vi "STS Calculator.vi"(8 "NumPts":i32=3, 10 "Saturation Id":dbl[](array[numeric]), 11 "Vg Column":dbl[](array[numeric])) -> (0 "STS Index":dbl, 2 "XY Graph":cluster{dbl[], dbl[]}[](graph), 3 "Sub Threshold Swing":dbl, 5 "Used Points":cluster{"Vg Used":dbl[], "Id Used":dbl[]})   [LabVIEW 2012]
uses:
  <vilib>/Analysis/NI_AALPro.lvlib
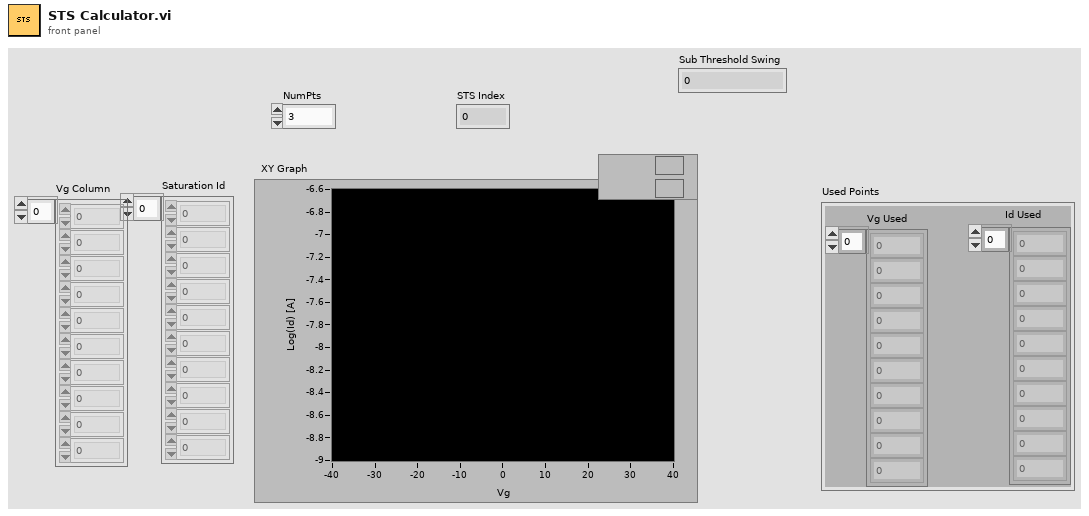
[diagram p1: front panel]
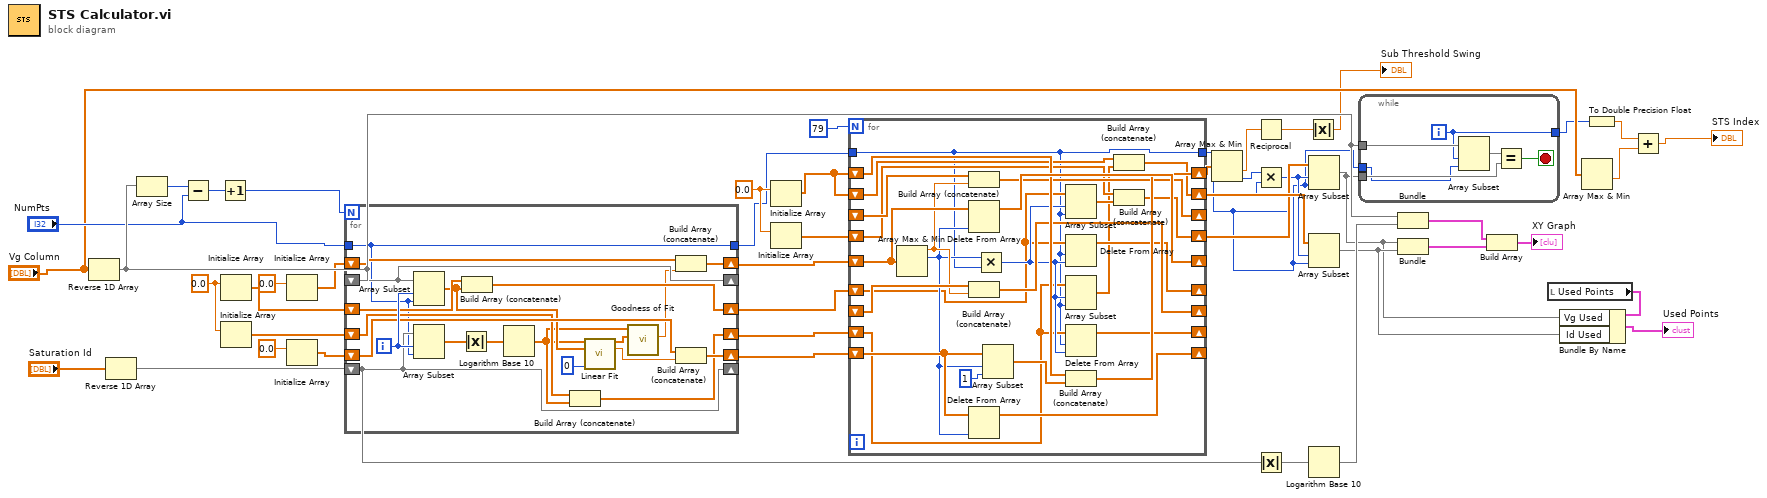
[diagram p0: block diagram]
diagram:
  w24 = 0.0
  w30 = 0.0
  n1 = Reverse 1D Array(array="Vg Column") -> (reversed array=w42:dbl[])
  n2 = Reverse 1D Array(array="Saturation Id") -> (reversed array=w11:dbl[])
  n3 = Array Size(array=w42) -> (size(s)=w41:i32)
  n4 = Subtract(x=w41, y="NumPts") -> (x-y=w17:i32)
  n5 = Increment(x=w17) -> (x+1=w16:i32)
  n6 = Initialize Array(w30) -> (w28:dbl[])  [unwired: 1 in]
  n7 = Initialize Array(w30) -> (w29:dbl[])  [unwired: 1 in]
  n8 = Initialize Array(0.0) -> (w39:dbl[])  [unwired: 1 in]
  n9 = Initialize Array(0.0) -> (w40:dbl[])  [unwired: 1 in]
  n10 = for {
    N: w16 -> [_]
    shift-right: [w54] -> _
    shift-left: w42 -> [w54]
    shift-right: [w60] -> _
    shift-left: w11 -> [w60]
    shift-right: [w64] -> w35
    shift-left: w40 -> [w63]
    shift-right: [w62] -> w33
    shift-left: w39 -> [w61]
    tunnel: "NumPts" -> [w47]
    shift-right: [w57] -> w27
    shift-left: w29 -> [w58]
    shift-right: [w55] -> w26
    shift-left: w28 -> [w56]
    tunnel: [w47] -> w7
    i -> [w66]
    n11 = Array Subset(array=w54, index=w66, length=w47) -> (w53:dbl[])
    n12 = Array Subset(array=w60, index=w66, length=w47) -> (w48:dbl[])
    n13 = Absolute Value(x=w48) -> (abs(x)=w49:dbl[])
    n14 = Build Array (concatenate)(w56, w53) -> (w55:dbl[])
    n15 = Logarithm Base 10(1:w49) -> (0:w50:dbl[])
    n16 = Build Array (concatenate)(w58, w50) -> (w57:dbl[])
    n17 = call <vilib>:"Linear Fit.vi"("Y"=w50, "X"=w53, "method"=0) -> ("Best Linear Fit"=w52:dbl[], "slope"=w65:dbl)  [unwired: 8 in, 3 out]
    n18 = call <vilib>:"Goodness of Fit.vi"("Best Fit"=w52, "Y"=w50) -> ("R-square"=w51:dbl)  [unwired: 6 in, 3 out]
    n19 = Build Array (concatenate)(w61, w51) -> (w62:dbl[])
    n20 = Build Array (concatenate)(w63, w65) -> (w64:dbl[])
  }
  n21 = Initialize Array(w24) -> (w20:dbl[])  [unwired: 1 in]
  n22 = Initialize Array(w24) -> (w25:dbl[])  [unwired: 1 in]
  n23 = for {
    N: 79 -> [_]
    shift-right: [w91] -> _
    shift-left: w33 -> [w92]
    shift-right: [w72] -> _
    shift-left: w35 -> [w73]
    shift-right: [w88] -> w34
    shift-left: w20 -> [w87]
    shift-right: [w86] -> _
    shift-left: _ -> [w85]
    shift-right: [w84] -> _
    shift-left: _ -> [w83]
    shift-right: [w82] -> _
    shift-left: w27 -> [w69]
    shift-right: [w80] -> _
    shift-left: w26 -> [w68]
    tunnel: w7 -> [w67]
    shift-right: [w79] -> w23
    shift-left: w20 -> [w78]
    shift-right: [w77] -> w22
    shift-left: w25 -> [w76]
    tunnel: [w67] -> w6
    n24 = Array Max & Min(array=w92) -> (max value=w71:dbl, max index (indices)=w70:i32)  [unwired: 2 out]
    n25 = Build Array (concatenate)(w83, w71) -> (w84:dbl[])
    n26 = Delete From Array(array=w92, index=w70) -> (array with subset deleted=w91:dbl[])  [unwired: 1 in, 1 out]
    n27 = Build Array (concatenate)(w85, w71) -> (w86:dbl[])
    n28 = Delete From Array(array=w73, index=w70) -> (array with subset deleted=w72:dbl[])  [unwired: 1 in, 1 out]
    n29 = Multiply(x=w70, y=w67) -> (x*y=w81:i32)
    n30 = Array Subset(array=w73, index=w70, length=1) -> (w89:dbl[])
    n31 = Array Subset(array=w68, index=w81, length=w67) -> (w75:dbl[])
    n32 = Delete From Array(array=w68, length=w67, index=w81) -> (array with subset deleted=w80:dbl[])  [unwired: 1 out]
    n33 = Array Subset(array=w69, index=w81, length=w67) -> (w74:dbl[])
    n34 = Delete From Array(array=w69, length=w67, index=w81) -> (array with subset deleted=w82:dbl[])  [unwired: 1 out]
    n35 = Build Array (concatenate)(w87, w89) -> (w88:dbl[])
    n36 = Build Array (concatenate)(w78, w74) -> (w79:dbl[])
    n37 = Build Array (concatenate)(w76, w75) -> (w77:dbl[])
  }
  n38 = Array Max & Min(array=w34) -> (min value=w45:dbl, min index (indices)=w21:i32)  [unwired: 2 out]
  n39 = Reciprocal(x=w45) -> (1/x=w46:dbl)
  n40 = Multiply(x=w21, y=w6) -> (x*y=w19:i32)
  n41 = Absolute Value(x=w11) -> (abs(x)=w44:dbl[])
  n42 = Absolute Value(x=w46) -> (abs(x)=→"Sub Threshold Swing":dbl)
  n43 = Array Subset(array=w22, index=w19, length=w6) -> (w13:dbl[])
  n44 = Array Subset(array=w23, index=w19, length=w6) -> (w14:dbl[])
  n45 = Logarithm Base 10(1:w44) -> (0:w43:dbl[])
  n46 = while {
    tunnel: w42 -> [w97]
    tunnel: w13 -> [w96]
    tunnel: [w94] -> w2
    tunnel: w6 -> [w93]
    i -> [w94]
    stop <- w98 stop-if-true
    n47 = Array Subset(array=w97, index=w94, length=w93) -> (w95:dbl[])
    n48 = Equal?(x=w95, y=w96) -> (x = y?=w98:bool)
  }
  n49 = Bundle(w42, w43) -> (w31:cluster{dbl[], dbl[]})  [unwired: 1 in]
  n50 = Bundle(w13, w14) -> (w18:cluster{dbl[], dbl[]})  [unwired: 1 in]
  n51 = Build Array(w31, w18) -> (→"XY Graph":cluster{dbl[], dbl[]}[])
  n52 = local read "Used Points"() -> (w15:cluster{"Vg Used":dbl[], "Id Used":dbl[]})
  n53 = Bundle By Name(cluster=w15, "Vg Used"=w13, "Id Used"=w14) -> (→"Used Points":cluster{"Vg Used":dbl[], "Id Used":dbl[]})
  n54 = Array Max & Min(array="Vg Column") -> (min value=w10:dbl)  [unwired: 3 out]
  n55 = To Double Precision Float(number=w2) -> (double precision float=w1:dbl)
  n56 = Add(x=w1, y=w10) -> (x+y=→"STS Index":dbl)
